vi "Keithley 2450 Read Backgate single.vi"(8 "error in (no error)":errorcluster, 11 "VISA resource name":refnum<visa-resource-name>) -> (0 "error out (no error) 2":errorcluster, 1 "Resistance (ohm)":dbl, 3 "VISA resource out":refnum<visa-resource-name>)   [LabVIEW 2019]
doc: "This example shows how to configure a measurement and take a reading."
uses:
  <instrlib>/Keithley 2450/Keithley 2450.lvlib
panel:
  out "read buffer":string
  out "Read Time":dbl
  out "Current (A)":dbl
  out "Voltage (V)":dbl
  # "(c) 2006 National Instruments.  ALL RIGHTS RESERVED."
  # "Source Settings"
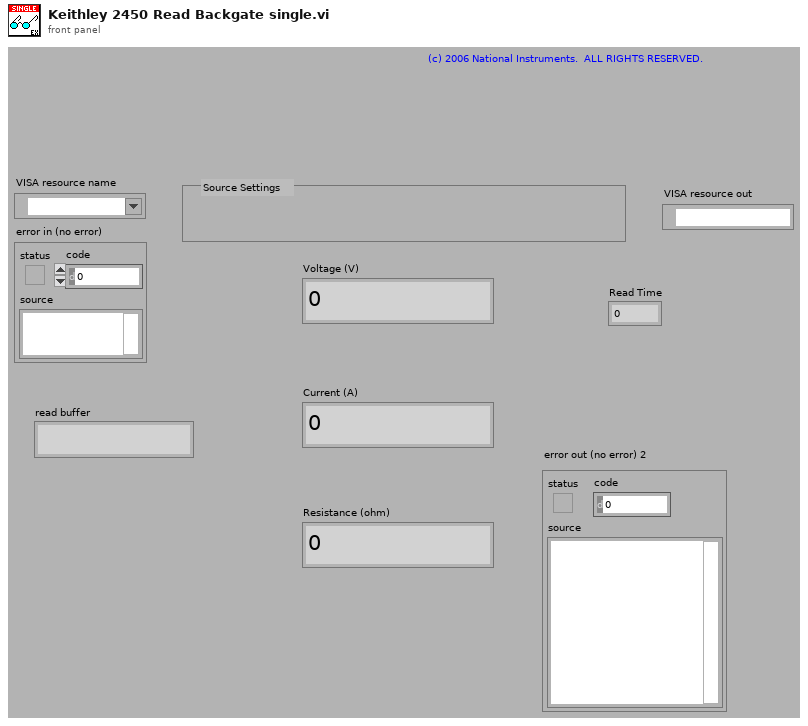
[diagram p1: front panel]
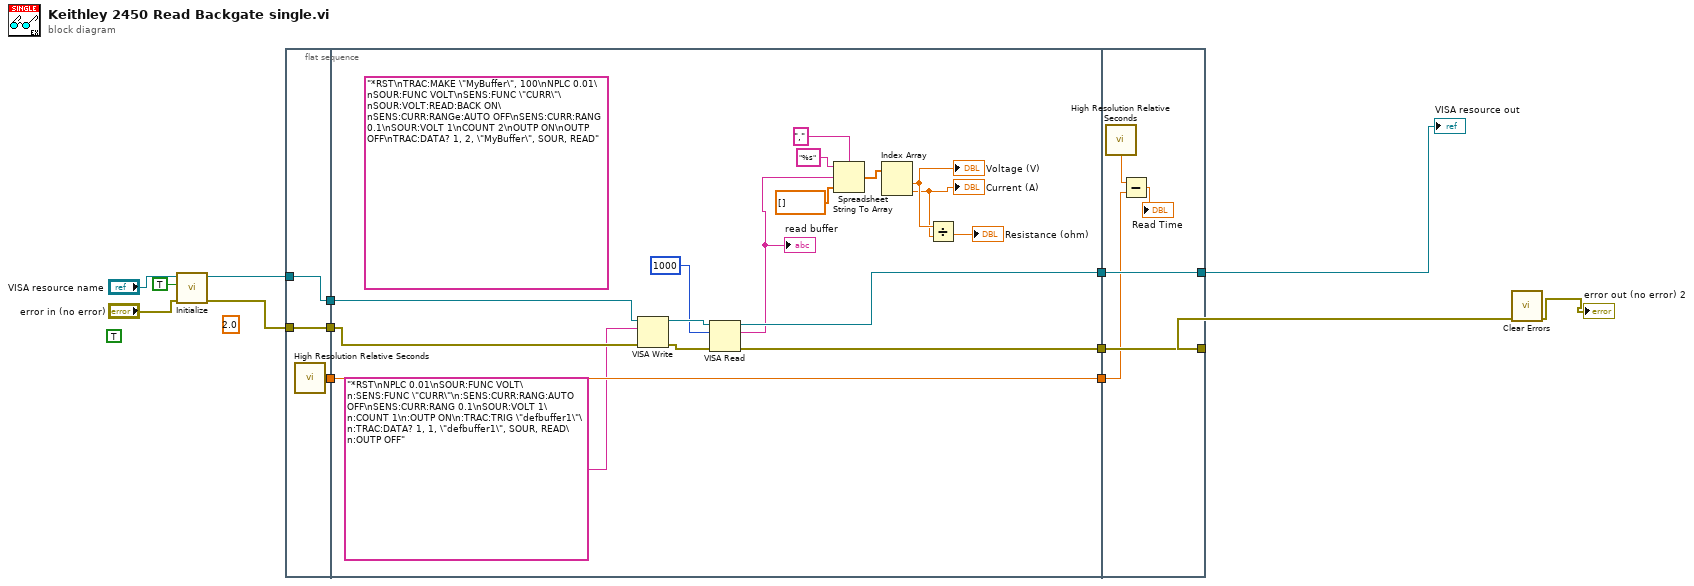
[diagram p0: block diagram]
diagram:
  (unwired) 2.0 ("Manual Range (1.0)")
  (unwired) TRUE ("Enable Output (T: Enable)")
  n1 = call <instrlib>:"Initialize.vi"("error in (no error)"="error in (no error)", "ID Query (True)"=TRUE, "VISA resource name"="VISA resource name") -> ("error out"=w7:errorcluster, "VISA resource name out"=w10:refnum<visa-resource-name>)  [unwired: 7 in]
  n2 = flat-sequence {
    tunnel: [w17] -> w11
    tunnel: w10 -> [w16]
    tunnel: [w16] -> w9
    tunnel: [w15] -> w8
    tunnel: w7 -> [w15]
    tunnel: w11 -> [w27]
    tunnel: w9 -> [w34]
    tunnel: w8 -> [w33]
    tunnel: [w29] -> w6
    tunnel: [w28] -> w5
    tunnel: [w27] -> w4
    tunnel: [w37] -> w3
    tunnel: w6 -> [w37]
    tunnel: w5 -> [w36]
    tunnel: [w36] -> w1
    tunnel: w4 -> [w35]
    frame #0 {
      n3 = call <vilib>:"High Resolution Relative Seconds.vi"() -> ("relative seconds"=w17:dbl)
    }
    frame #1 {
      (unwired) "*RST\nTRAC:MAKE \"MyBuffer\", 100\nNPLC 0.01\nSOUR:FUNC VOLT\nSENS:FUNC \"CURR\"\nSOUR:VOLT:READ:BACK ON\nSENS:CURR:RANGe:AUTO OFF\nSENS:CURR:RANG 0.1\nSOUR:VOLT 1\nCOUNT 2\nOUTP ON\nOUTP OFF\nTRAC:DATA? 1, 2, \"MyBuffer\", SOUR, READ" ("write buffer")
      n4 = VISA Write(VISA resource name=w34, write buffer="*RST\nNPLC 0.01\nSOUR:FUNC VOLT\n:SENS:FUNC \"CURR\"\n:SENS:CURR:RANG:AUTO OFF\nSENS:CURR:RANG 0.1\nSOUR:VOLT 1\n:COUNT 1\n:OUTP ON\n:TRAC:TRIG \"defbuffer1\"\n:TRAC:DATA? 1, 1, \"defbuffer1\", SOUR, READ\n:OUTP OFF", error in (no error)=w33) -> (VISA resource name out=w32:refnum<visa-resource-name>, error out=w31:errorcluster)  [unwired: 1 out]
      n5 = VISA Read(VISA resource name=w32, byte count=u32 1000, error in (no error)=w31) -> (VISA resource name out=w29:refnum<visa-resource-name>, read buffer=w24:string, error out=w28:errorcluster)  [unwired: 1 out]
      "read buffer" <- w24
      n6 = Spreadsheet String To Array(delimiter (Tab)=",", format string="%s", spreadsheet string=w24, array type (2D Dbl)=dbl[] []) -> (array=w22:dbl[])
      n7 = Index Array(array=w22) -> (element #1=w20:dbl, element #2=w19:dbl)  [unwired: 2 in]
      "Voltage (V)" <- w20
      "Current (A)" <- w19
      n8 = Divide(x=w20, y=w19) -> (x/y=→"Resistance (ohm)":dbl)
    }
    frame #2 {
      n9 = call <vilib>:"High Resolution Relative Seconds.vi"() -> ("relative seconds"=w39:dbl)
      n10 = Subtract(x=w39, y=w35) -> (x-y=→"Read Time":dbl)
    }
  }
  n11 = call <vilib>:"Clear Errors.vi"("error in (no error)"=w1) -> ("error out"=→"error out (no error) 2":errorcluster)  [unwired: 5 in, 1 out]
  "VISA resource out" <- w3
